vi "Updated Route.vi"(8 "New position":i32[](array[numeric]), 9 "New element":string, 10 "Route":i32[][](array[numeric]), 11 "Current element":string) -> (2 "Can move":bool, 3 "Updated Route":i32[][](array[numeric]))   [LabVIEW 2021]
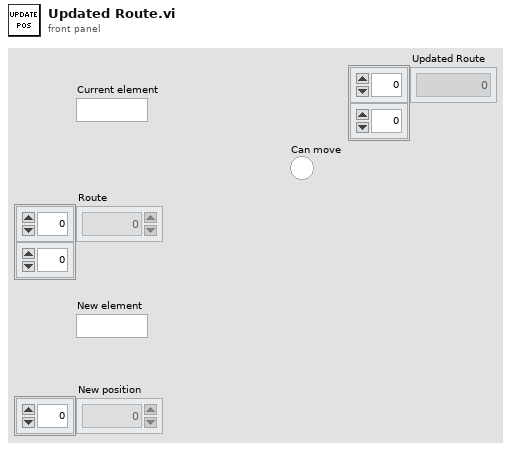
[diagram p1: front panel]
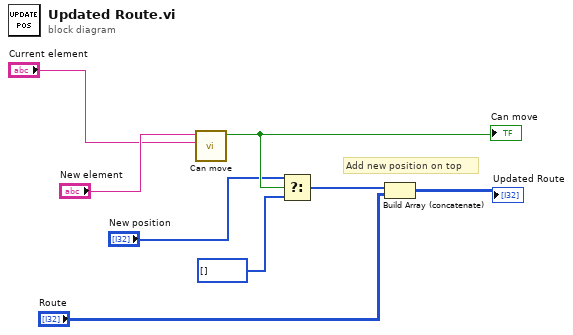
[diagram p0: block diagram]
diagram:
  # "Add new position on top"
  n1 = call "Can move"("Current letter"="Current element", "New letter"="New element") -> ("Can move"=w5:bool)  [unwired: 9 in]
  "Can move" <- w5
  n2 = Select(t="New position", s=w5, f=i32[] []) -> (s? t:f=w7:i32[])
  n3 = Build Array (concatenate)(w7, "Route") -> (→"Updated Route":i32[][])
